vi "__del__.vi"(8 "error in":errorcluster, 11 "Resonance Curve in":refnum<class "Resonance Curve.lvclass">) -> ()   [LabVIEW 2020, in "Resonance Curve.lvclass"]
uses:
  Resonance Curve.lvclass
  Resonance Curve.lvclass/Resonance Curve.ctl
  Function Generator/Function Generator.lvclass
  Lock-In Amplifier/Lock-In Amplifier.lvclass
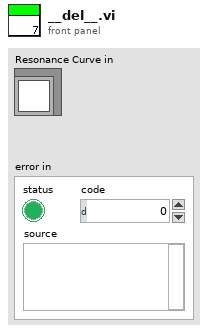
[diagram p1: front panel]
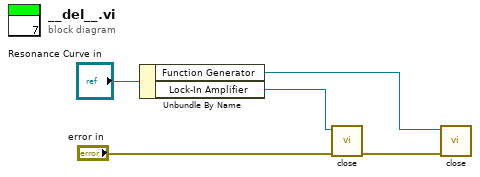
[diagram p0: block diagram]
diagram:
  n1 = Unbundle By Name("Resonance Curve in") -> ("Function Generator"=w4:refnum<class "Function Generator.lvclass">, "Lock-In Amplifier"=w3:refnum<class "Lock-In Amplifier.lvclass">)
  n2 = call-dynamic "close.vi"("error in (no error)"="error in", "Instrument in"=w3) -> ("error out"=w2:errorcluster)  [unwired: 9 in]
  n3 = call-dynamic "close.vi"("error in (no error)"=w2, "Function Generator in"=w4) -> ()  [unwired: 9 in, 1 out]
